vi "Send RegisterAppenderMsg.vi"(8 "error in (no error)":errorcluster, 10 "Lumberjack.lvlib:Appender.lvclass":refnum<class "Appender.lvclass">, 11 "Enqueuer in":refnum<class "Message Enqueuer.lvclass">) -> (0 "error out":errorcluster, 3 "Enqueuer out":refnum<class "Message Enqueuer.lvclass">)   [LabVIEW 2026, in "Lumberjack.lvlib" / "RegisterAppenderMsg.lvclass"]
doc: "Construct a RegisterAppenderMsg carrying a configured Appender and enqueue it to the LogManager. The manager's Do launches the appender as a nested actor, registers it, and posts an updated Snapshot. Called by the Logger's add-appender control wrapper (SRS-LMBR-045)."
uses:
  RegisterAppenderMsg.lvclass
  <vilib>/ActorFramework/Message Enqueuer/Message Enqueuer.lvclass
  Appenders/Appender.lvclass/Appender.lvclass
  RegisterAppenderMsg.lvclass/RegisterAppenderMsg.ctl
  <vilib>/ActorFramework/Message Enqueuer/Message Enqueuer.lvclass/Message Enqueuer.ctl
  <vilib>/ActorFramework/Message Priority Queue/Priority Enqueue.vi
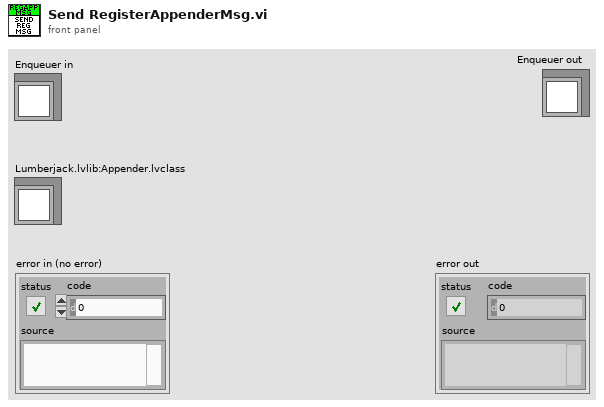
[diagram p1: front panel]
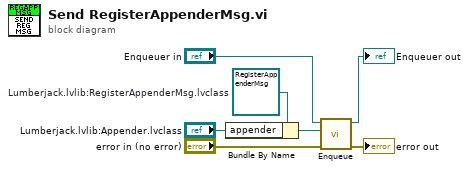
[diagram p0: block diagram]
diagram:
  w3 = refnum<class "RegisterAppenderMsg.lvclass"> refnum  # Lumberjack.lvlib:RegisterAppenderMsg.lvclass
  n1 = Bundle By Name(cluster=w3, "appender"="Lumberjack.lvlib:Appender.lvclass") -> (w2:refnum<class "RegisterAppenderMsg.lvclass">)
  n2 = call <vilib>:"Enqueue.vi"("error in (no error)"="error in (no error)", "Message"=w2, "Message Enqueuer in"="Enqueuer in") -> ("error out"=→"error out":errorcluster, "Message Enqueuer out"=→"Enqueuer out":refnum<class "Message Enqueuer.lvclass">)  [unwired: 7 in]
